vi "ImageListDemo.vi"   [LabVIEW 2012]
uses:
  System.Windows.Forms
  System.Drawing
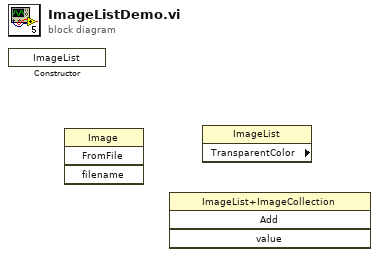
[diagram p0: block diagram]
diagram:
  n1 = constructor class="ImageList"() -> ()  [unwired: 3 in, 3 out]
  n2 = invoke class="Image" method="FromFile"() -> ()  [unwired: 4 in, 4 out]
  n3 = invoke class="ImageList+ImageCollection" method="Add"() -> ()  [unwired: 4 in, 4 out]
  n4 = property class="ImageList" props=["TransparentColor"]() -> ()  [unwired: 2 in, 3 out]
